vi "HexCenterFinder6Points.vi"() -> ()   [LabVIEW 2019]
uses:
  <vilib>/userDefined/High Color/IMAQdx.ctl
  <vilib>/vision/NI_Vision_Development_Module.lvlib
panel:
  in  "VisibleCorners":bool
  in  "AdjustCamera":T1={"+Y"=FALSE, "-Z"=FALSE, "Done"=FALSE, "+Z"=FALSE, "-Y"=FALSE, "-X"=FALSE, "+X"=FALSE, "MoveXYBy(mm)"=0.25, "MoveZBy(mm)"=0.1} {"MoveZBy(mm)" format="%#_13g"}
  out "CameraGcode":string
  out "Gcode":string
  out "Image":T2(plugin-control)
  in  "SiPatternLocations":path=path "C:/Users/TTUHEP/Documents/LabVIEW/Data/AssemblyIO_logs/Si2Fiducials.txt"
  out "Dev":dbl
  in  "YoffsetPCB":dbl format="%#_13g"
  in  "XoffsetPCB":dbl format="%#_13g"
  in  "Position1?":bool=TRUE
  in  "Yoffset":dbl format="%#_13g"
  in  "Xoffset":dbl=165.962 format="%#_13g"
  out "Output XYZU":string
  in  "PCBEdges":path=path "C:/Users/TTUHEP/Documents/LabVIEW/Data/AssemblyIO_logs/PCB1_4Points.txt"
  in  "SiNoPatternCorners":path=path "C:/Users/TTUHEP/Documents/LabVIEW/Data/AssemblyIO_logs/Si2Corners.txt"
  in  "Component":T3(ring)
  in  "BasePlateEdges":path=path "C:/Users/TTUHEP/Documents/LabVIEW/Data/AssemblyIO_logs/Baseplate1CuPoints.txt"
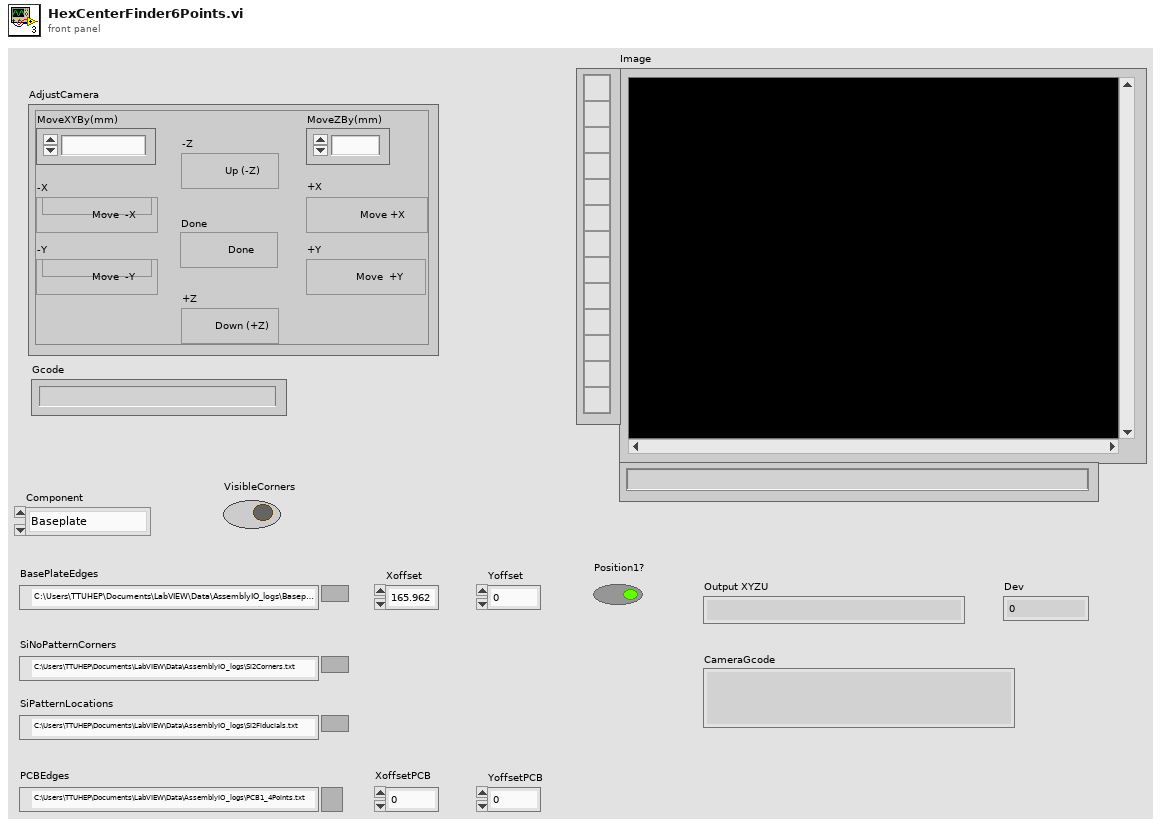
[diagram p1: front panel]
types:
  T1 = cluster{"+Y":bool, "-Z":bool, "Done":bool, "+Z":bool, "-Y":bool, "-X":bool, "+X":bool, "MoveXYBy(mm)":dbl, "MoveZBy(mm)":dbl}
  T2 = typedef "IMAQ Image.ctl" = refnum<image>
  T3 = enum16{"Baseplate", "SiNoPattern", "SiPattern", "PCB"}
  T4 = typedef "IMAQdx.ctl" = refnum<k21>
  T5 = typedef "IMAQ Point" = cluster{"X":sgl, "Y":sgl}
  T6 = enum16{"Left Button", "Center Button", "Right Button", "Window Close"}
  T7 = enum16{"open", "replace", "create", "open or create", "replace or create", "replace or create with confirmation"}
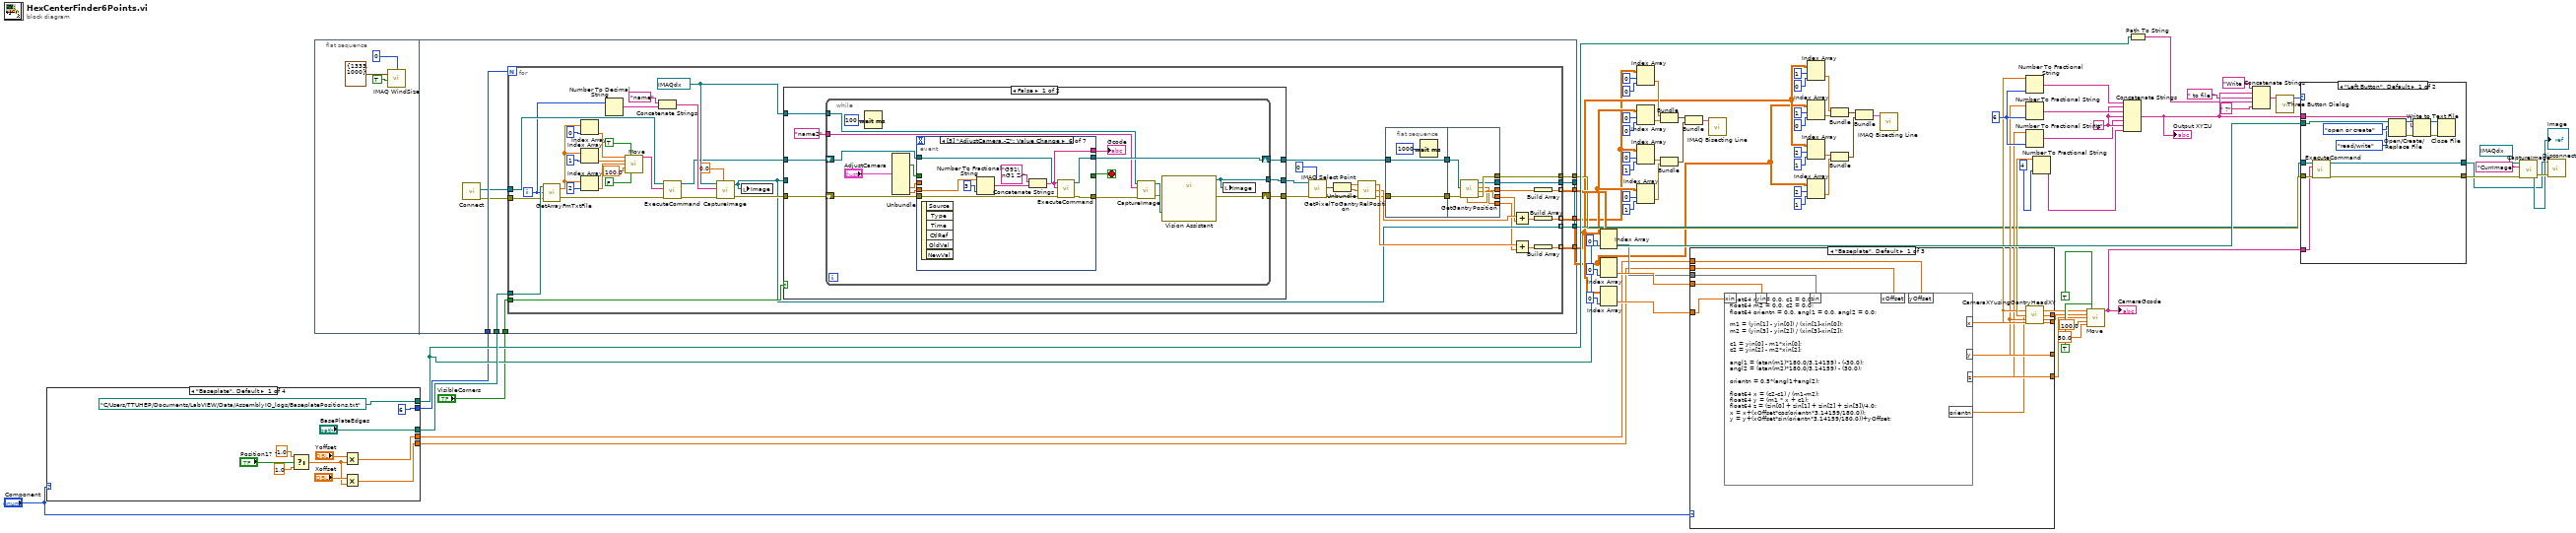
[diagram p0: block diagram]
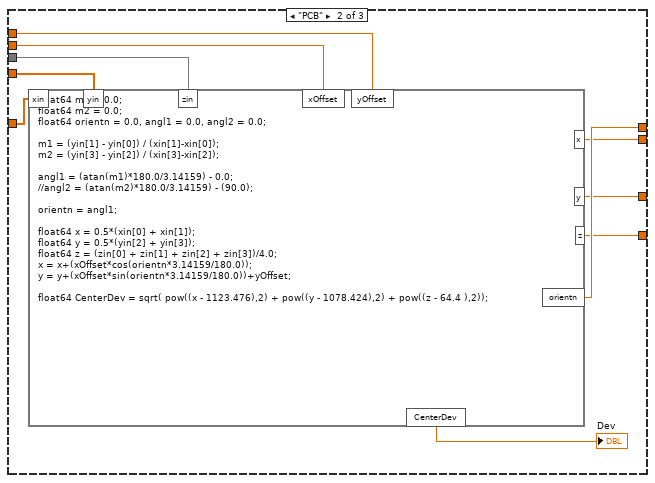
[diagram p2: hidden frame]
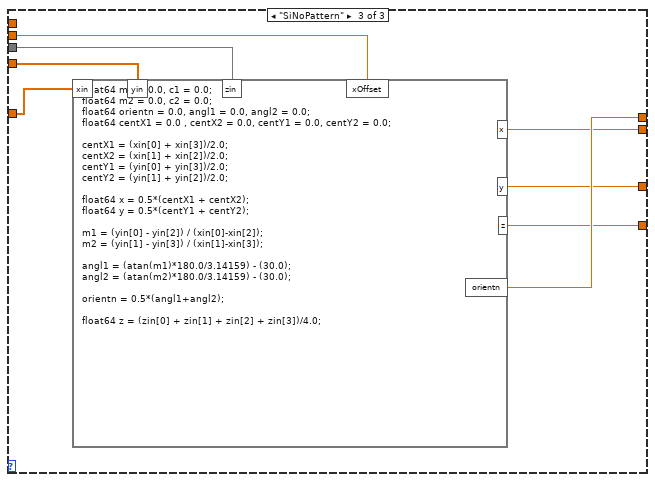
[diagram p3: hidden frame]
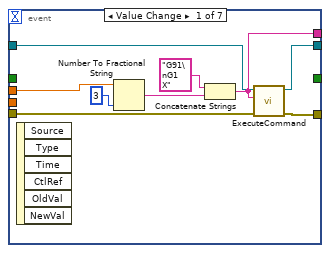
[diagram p5: hidden frame]
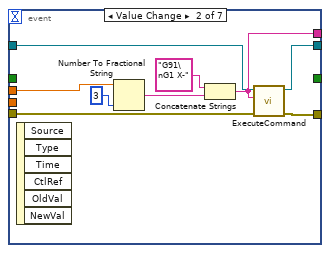
[diagram p6: hidden frame]
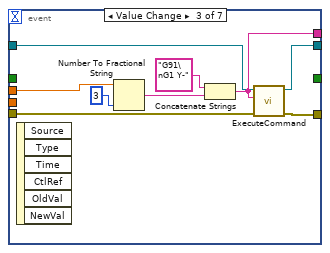
[diagram p7: hidden frame]
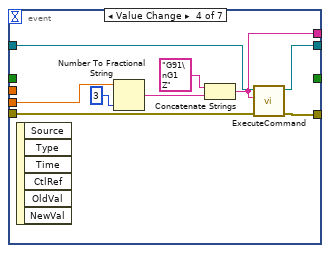
[diagram p8: hidden frame]
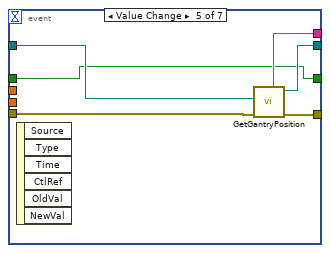
[diagram p9: hidden frame]
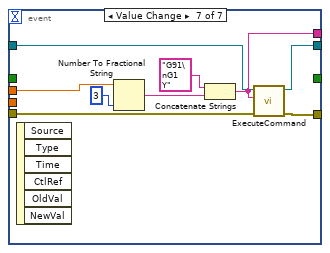
[diagram p10: hidden frame]
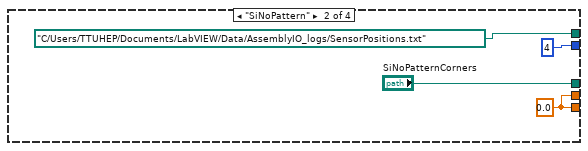
[diagram p12: hidden frame]
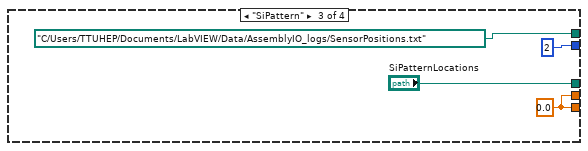
[diagram p13: hidden frame]
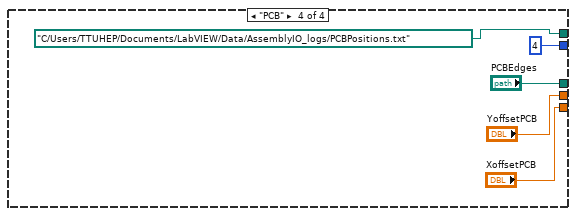
[diagram p14: hidden frame]
diagram:
  w76 = "\t"
  w73 = i16 6 ("width (-)")
  n1 = case shown="\"Baseplate\", Default" "Component" {
    tunnel: ["BasePlateEdges" "SiNoPatternCorners" "SiPatternLocations" "PCBEdges"] -> w79
    tunnel: [path "C:/Users/TTUHEP/Documents/LabVIEW/Data/AssemblyIO_logs/BaseplatePositions.txt" ("OutFile") path "C:/Users/TTUHEP/Documents/LabVIEW/Data/AssemblyIO_logs/SensorPositions.txt" ("OutFile") path "C:/Users/TTUHEP/Documents/LabVIEW/Data/AssemblyIO_logs/SensorPositions.txt" ("OutFile") path "C:/Users/TTUHEP/Documents/LabVIEW/Data/AssemblyIO_logs/PCBPositions.txt" ("OutFile")] -> w64
    tunnel: [w82 w92 w96 "YoffsetPCB"] -> w54
    tunnel: [w81 w92 w96 "XoffsetPCB"] -> w53
    tunnel: [6 4 2 4] -> w40
    frame "Baseplate", Default {
      n2 = Select(t=-1.0, s="Position1?", f=1.0 ("t")) -> (s? t:f=w83:dbl)
      n3 = Multiply(x="Yoffset", y=w83) -> (x*y=w82:dbl)
      n4 = Multiply(x="Xoffset", y=w83) -> (x*y=w81:dbl)
    }
    frame "SiNoPattern" {
      w92 = 0.0 ("YoffsetPCB")
    }
    frame "SiPattern" {
      w96 = 0.0 ("XoffsetPCB")
    }
    frame "PCB" {
    }
  }
  n5 = flat-sequence {
    tunnel: w40 -> [w117]
    tunnel: w79 -> [w116]
    tunnel: [w115] -> w38
    tunnel: [w114] -> w36
    tunnel: [w111] -> _
    tunnel: [w110] -> w62
    tunnel: [w109] -> w1
    tunnel: [w108] -> w2
    tunnel: "VisibleCorners" -> [w107]
    frame #0 {
      n6 = call "IMAQ WindSize"("Scrollbars? (N)"=TRUE, "Width & Height"=cluster{"Width":i32, "Height":i32} {"Width"=1333, "Height"=1000}, "Window Number"=0) -> ()  [unwired: 3 in, 3 out]
    }
    frame #1 {
      n7 = call "Connect.vi"() -> ("error out"=w113:errorcluster, "controller"=w112:refnum<k24>)  [unwired: 10 in]
      n8 = for {
        N: w117 -> [_]
        tunnel: w116 -> [w162]
        tunnel: w112 -> [w155]
        tunnel: w113 -> [w154]
        tunnel: [w126] -> w115
        tunnel: [w123] -> w114
        tunnel: [w127] -> w111 mode=indexing
        tunnel: [w148] -> w110 mode=indexing
        tunnel: [w142] -> w109 mode=indexing
        tunnel: [w141] -> w108 mode=indexing
        tunnel: w107 -> [w128]
        i -> [w152]
        w133 = T4 "cam0" ("Camera")
        n9 = call "GetArrayFmTxtFile.vi"("error in"=w154, "LineNo."=w152, "TextFile"=w162) -> ("error out"=w153:errorcluster, "Array"=w163:dbl[])
        n10 = Index Array(array=w163, index=0) -> (element=w139:dbl)
        n11 = Index Array(array=w163, index=1) -> (element=w137:dbl)
        n12 = Index Array(array=w163, index=2) -> (element=w147:dbl)
        n13 = Number To Decimal String(number=w152) -> (decimal integer string=w151:string)  [unwired: 1 in]
        n14 = call "Move.vi"("X"=w139, "Absolute"=TRUE, "Y"=w137, "Z"=w147, "SpeedXY (mm/s)"=100.0, "Move Z first"=FALSE) -> ("Position Gcode"=w156:string)  [unwired: 9 in]
        n15 = Concatenate Strings("name" ("string"), w151) -> (w149:string)
        n16 = call "ExecuteCommand.vi"("error in (no error)"=w153, "Command Code"=w156, "controller in"=w155) -> ("error out"=w158:errorcluster, "controller out"=w132:refnum<k24>)  [unwired: 6 in, 1 out]
        n17 = call "CaptureImage.vi"("Camera"=w133, "Rotate (degrees)"=sgl 0.0, "ImageName"=w149, "error in (no error)"=w158) -> ("Image"=w127:T2, "error out"=w131:errorcluster)  [unwired: 3 in]
        n18 = local write "Image"(w127) -> ()
        n19 = case shown="False" w128 {
          tunnel: w133 -> [w182 _]
          tunnel: w132 -> [w181 w262]
          tunnel: w131 -> [w180 w263]
          tunnel: [w179 w261] -> w130
          tunnel: [w178 w262] -> w119
          tunnel: [w177 w263] -> w129
          tunnel: w127 -> [_ w261]
          frame False {
            n20 = while {
              shift-right: [w191] -> w177
              shift-left: w180 -> [w200]
              shift-right: [w198] -> w178
              shift-left: w181 -> [w199]
              tunnel: "name2" ("ImageName") -> [w193]
              tunnel: w182 -> [w194]
              tunnel: [w190] -> w179
              stop <- w196 stop-if-true
              n21 = Wait (ms)(milliseconds to wait=u32 100) -> ()  [unwired: 1 out]
              n22 = Unbundle("AdjustCamera") -> ("Done"=w186:bool, "MoveXYBy(mm)"=w184:dbl, "MoveZBy(mm)"=w185:dbl)  [unwired: 6 out]
              n23 = event shown="[5] \"AdjustCamera.-Z\": Value Change" {
                selector: _ -> [_ _ _ _ _ _ _]
                dyn-events: _ -> [_ _ _ _ _ _ _]
                timeout: _ -> [_ _ _ _ _ _ _]
                tunnel: w184 -> [w206 w210 w219 _ _ _ w252]
                tunnel: w200 -> [w205 w214 w223 w232 w241 w247 w256]
                tunnel: [w204 w213 w222 w229 w238 w246 w255] -> w192
                tunnel: w199 -> [w203 w215 w224 w233 w242 w248 w257]
                tunnel: [w202 w212 w221 w230 w240 w245 w254] -> w198
                tunnel: [w201 w211 w220 w231 w239 w244 w253] -> w197
                tunnel: [_ _ _ _ w237 _ _] -> w196
                tunnel: w185 -> [_ _ _ w228 _ w243 _]
                tunnel: w186 -> [_ _ _ _ w237 _ _]
                event "AdjustCamera.+X": Value Change {
                  n24 = event-data() -> ()  [unwired: 1 in, 6 out]
                  n25 = Number To Fractional String(number=w206, precision (6)=3) -> (F-format string=w209:string)  [unwired: 2 in]
                  n26 = Concatenate Strings("G91\nG1 X", w209) -> (w201:string)
                  n27 = call "ExecuteCommand.vi"("error in (no error)"=w205, "Command Code"=w201, "controller in"=w203) -> ("error out"=w204:errorcluster, "controller out"=w202:refnum<k24>)  [unwired: 6 in, 1 out]
                }
                event "AdjustCamera.-X": Value Change {
                  n28 = event-data() -> ()  [unwired: 1 in, 6 out]
                  n29 = Number To Fractional String(number=w210, precision (6)=3) -> (F-format string=w218:string)  [unwired: 2 in]
                  n30 = Concatenate Strings("G91\nG1 X-", w218) -> (w211:string)
                  n31 = call "ExecuteCommand.vi"("error in (no error)"=w214, "Command Code"=w211, "controller in"=w215) -> ("error out"=w213:errorcluster, "controller out"=w212:refnum<k24>)  [unwired: 6 in, 1 out]
                }
                event "AdjustCamera.-Y": Value Change {
                  n32 = event-data() -> ()  [unwired: 1 in, 6 out]
                  n33 = Number To Fractional String(number=w219, precision (6)=3) -> (F-format string=w227:string)  [unwired: 2 in]
                  n34 = Concatenate Strings("G91\nG1 Y-", w227) -> (w220:string)
                  n35 = call "ExecuteCommand.vi"("error in (no error)"=w223, "Command Code"=w220, "controller in"=w224) -> ("error out"=w222:errorcluster, "controller out"=w221:refnum<k24>)  [unwired: 6 in, 1 out]
                }
                event "AdjustCamera.+Z": Value Change {
                  n36 = event-data() -> ()  [unwired: 1 in, 6 out]
                  n37 = Number To Fractional String(number=w228, precision (6)=3) -> (F-format string=w236:string)  [unwired: 2 in]
                  n38 = Concatenate Strings("G91\nG1 Z", w236) -> (w231:string)
                  n39 = call "ExecuteCommand.vi"("error in (no error)"=w232, "Command Code"=w231, "controller in"=w233) -> ("error out"=w229:errorcluster, "controller out"=w230:refnum<k24>)  [unwired: 6 in, 1 out]
                }
                event "AdjustCamera.Done": Value Change {
                  n40 = event-data() -> ()  [unwired: 1 in, 6 out]
                  n41 = call "GetGantryPosition.vi"("error in (no error)"=w241, "Controller In"=w242) -> ("error out"=w238:errorcluster, "controller out"=w240:refnum<k24>, "Position_XYZ"=w239:string)  [unwired: 3 in, 4 out]
                }
                event "AdjustCamera.-Z": Value Change {
                  n42 = event-data() -> ()  [unwired: 1 in, 6 out]
                  n43 = Number To Fractional String(number=w243, precision (6)=3) -> (F-format string=w251:string)  [unwired: 2 in]
                  n44 = Concatenate Strings("G91\nG1 Z-", w251) -> (w244:string)
                  n45 = call "ExecuteCommand.vi"("error in (no error)"=w247, "Command Code"=w244, "controller in"=w248) -> ("error out"=w246:errorcluster, "controller out"=w245:refnum<k24>)  [unwired: 6 in, 1 out]
                }
                event "AdjustCamera.+Y": Value Change {
                  n46 = event-data() -> ()  [unwired: 1 in, 6 out]
                  n47 = Number To Fractional String(number=w252, precision (6)=3) -> (F-format string=w260:string)  [unwired: 2 in]
                  n48 = Concatenate Strings("G91\nG1 Y", w260) -> (w253:string)
                  n49 = call "ExecuteCommand.vi"("error in (no error)"=w256, "Command Code"=w253, "controller in"=w257) -> ("error out"=w255:errorcluster, "controller out"=w254:refnum<k24>)  [unwired: 6 in, 1 out]
                }
              }
              "Gcode" <- w197
              n50 = call "CaptureImage.vi"("Camera"=w194, "ImageName"=w193, "error in (no error)"=w192) -> ("Image"=w189:T2, "error out"=w188:errorcluster)  [unwired: 4 in]
              n51 = call "Vision Assistant"("Image In"=w189, "error in"=w188) -> ("Image Out"=w190:T2, "error out"=w191:errorcluster)  [unwired: 24 in]
              n52 = local write "Image"(w190) -> ()
            }
          }
          frame True {
          }
        }
        n53 = call "IMAQ Select Point"("Window Number (0...15)"=0, "error in (no error)"=w129, "Image In"=w130) -> ("error out"=w143:errorcluster, "Point"=w146:T5)  [unwired: 5 in, 2 out]
        n54 = Unbundle(w146) -> ("X"=w145:sgl, "Y"=w144:sgl)
        n55 = call "GetPixelToGantryRelPosition.vi"("error in (no error)"=w143, "PixelY"=w144, "PixelX"=w145) -> ("error out"=w121:errorcluster, "YmmRelGH"=w136:dbl, "XmmRelGH"=w140:dbl)
        n56 = flat-sequence {
          tunnel: w121 -> [w168]
          tunnel: [w168] -> w120
          tunnel: w119 -> [w167]
          tunnel: [w167] -> w118
          tunnel: [w176] -> w126
          tunnel: [w175] -> w125
          tunnel: [w174] -> w124
          tunnel: [w173] -> w123
          tunnel: [w172] -> w122
          tunnel: w120 -> [w171]
          tunnel: w118 -> [w170]
          frame #0 {
            n57 = Wait (ms)(milliseconds to wait=u32 1000) -> ()  [unwired: 1 out]
          }
          frame #1 {
            n58 = call "GetGantryPosition.vi"("error in (no error)"=w171, "Controller In"=w170) -> ("error out"=w176:errorcluster, "Position Y"=w175:dbl, "Position X"=w174:dbl, "controller out"=w173:refnum<k24>, "Position Z"=w172:dbl)  [unwired: 3 in, 2 out]
          }
        }
        n59 = Add(x=w136, y=w125) -> (x+y=w135:dbl)
        n60 = Add(x=w140, y=w124) -> (x+y=w138:dbl)
        n61 = Build Array(w122) -> (w148:dbl[])
        n62 = Build Array(w135) -> (w142:dbl[])
        n63 = Build Array(w138) -> (w141:dbl[])
      }
    }
  }
  n64 = Index Array(array=w62, index (col)=0 ("disabled index (col)")) -> (element=w57:dbl[])  [unwired: 1 in]
  n65 = Index Array(array=w1, index (col)=0 ("disabled index (col)")) -> (element=w58:dbl[])  [unwired: 1 in]
  n66 = Index Array(array=w2, index (col)=0 ("disabled index (col)")) -> (element=w59:dbl[])  [unwired: 1 in]
  n67 = Index Array(array=w1, index (row)=0 ("disabled index (row)"), index (col)=0 ("disabled index (col)")) -> (element=w24:dbl)
  n68 = Index Array(array=w2, index (row)=0 ("disabled index (row)"), index (col)=0 ("disabled index (col)")) -> (element=w23:dbl)
  n69 = Index Array(array=w1, index (row)=0 ("disabled index (row)"), index (col)=1 ("disabled index (col)")) -> (element=w22:dbl)
  n70 = Index Array(array=w2, index (row)=0 ("disabled index (row)"), index (col)=1 ("disabled index (col)")) -> (element=w21:dbl)
  n71 = Bundle(w24, w23) -> (w20:cluster{dbl, dbl})  [unwired: 1 in]
  n72 = Bundle(w22, w21) -> (w19:cluster{dbl, dbl})  [unwired: 1 in]
  n73 = Bundle(w20, w19) -> (w18:cluster{cluster{dbl, dbl}, cluster{dbl, dbl}})  [unwired: 1 in]
  n74 = case shown="\"Baseplate\", Default" "Component" {
    tunnel: w59 -> [w272 w282 w290]
    tunnel: w58 -> [w271 w281 w289]
    tunnel: w57 -> [w270 w280 w288]
    tunnel: w53 -> [w269 w279 w287]
    tunnel: [w268 w278 w286] -> w56
    tunnel: [w267 w277 w285] -> w45
    tunnel: [w266 w276 w284] -> w44
    tunnel: [w265 w275 w283] -> w41
    tunnel: w54 -> [w264 w274 _]
    frame "Baseplate", Default {
      n75 = formula code="float64 m1 = 0.0, c1 = 0.0;\nfloat64 m2 = 0.0, c2 = 0.0;\nfloat64 orientn = 0.0, angl1 = 0.0, angl2 = 0.0;\n\nm1 = (yin[1] - yin[0]) / (xin[1]-xin[0]);\nm2 = (yin[3] - yin[2]) / (xin[3]-xin[2]);\n\nc1 = yin[0] - m1*xin[0];\nc2 = yin[2] - m2*xin[2];\n\nangl1 = (atan(m1)*180.0/3.14159) - (-30.0);\nangl2 = (atan(m2)*180.0/3.14159) - (30.0);\n\norientn = 0.5*(angl1+angl2);\n\nfloat64 x = (c2-c1) / (m1-m2);\nfloat64 y = (m1 * x + c1);\nfloat64 z = (zin[0] + zin[1] + zin[2] + zin[3])/4.0;\nx = x+(xOffset*cos(orientn*3.14159/180.0));\ny = y+(xOffset*sin(orientn*3.14159/180.0))+yOffset;"("xin"=w272, "yin"=w271, "zin"=w270, "xOffset"=w269, "yOffset"=w264) -> ("orientn"=w268:dbl, "x"=w267:dbl, "y"=w266:dbl, "z"=w265:dbl)
    }
    frame "PCB" {
      n76 = formula code="float64 m1 = 0.0;\nfloat64 m2 = 0.0;\nfloat64 orientn = 0.0, angl1 = 0.0, angl2 = 0.0;\n\nm1 = (yin[1] - yin[0]) / (xin[1]-xin[0]);\nm2 = (yin[3] - yin[2]) / (xin[3]-xin[2]);\n\nangl1 = (atan(m1)*180.0/3.14159) - 0.0;\n//angl2 = (atan(m2)*180.0/3.14159) - (90.0);\n\norientn = angl1;\n\nfloat64 x = 0.5*(xin[0] + xin[1]);\nfloat64 y = 0.5*(yin[2] + yin[3]);\nfloat64 z = (zin[0] + zin[1] + zin[2] + zin[3])/4.0;\nx = x+(xOffset*cos(orientn*3.14159/180.0));\ny = y+(xOffset*sin(orientn*3.14159/180.0))+yOffset;\n\nfloat64 CenterDev = sqrt( pow((x - 1123.476),2) + pow((y - 1078.424),2) + pow((z - 64.4 ),2));"("xin"=w282, "yin"=w281, "zin"=w280, "xOffset"=w279, "yOffset"=w274) -> ("orientn"=w278:dbl, "x"=w277:dbl, "y"=w276:dbl, "z"=w275:dbl, "CenterDev"=→"Dev":dbl)
    }
    frame "SiNoPattern" {
      n77 = formula code="float64 m1 = 0.0, c1 = 0.0;\nfloat64 m2 = 0.0, c2 = 0.0;\nfloat64 orientn = 0.0, angl1 = 0.0, angl2 = 0.0;\nfloat64 centX1 = 0.0 , centX2 = 0.0, centY1 = 0.0, centY2 = 0.0;\n\ncentX1 = (xin[0] + xin[3])/2.0;\ncentX2 = (xin[1] + xin[2])/2.0;\ncentY1 = (yin[0] + yin[3])/2.0;\ncentY2 = (yin[1] + yin[2])/2.0;\n\nfloat64 x = 0.5*(centX1 + centX2); \nfloat64 y = 0.5*(centY1 + centY2);\n\nm1 = (yin[0] - yin[2]) / (xin[0]-xin[2]);\nm2 = (yin[1] - yin[3]) / (xin[1]-xin[3]);\n\nangl1 = (atan(m1)*180.0/3.14159) - (30.0);\nangl2 = (atan(m2)*180.0/3.14159) - (30.0);\n\norientn = 0.5*(angl1+angl2);\n\nfloat64 z = (zin[0] + zin[1] + zin[2] + zin[3])/4.0;"("xin"=w290, "yin"=w289, "zin"=w288, "xOffset"=w287) -> ("orientn"=w286:dbl, "x"=w285:dbl, "y"=w284:dbl, "z"=w283:dbl)
    }
  }
  n78 = call "IMAQ Bisecting Line"("Line 1"=w18) -> ()  [unwired: 9 in, 2 out]
  n79 = Index Array(array=w2, index (row)=1 ("disabled index (row)"), index (col)=0 ("disabled index (col)")) -> (element=w9:dbl)
  n80 = Index Array(array=w1, index (row)=1 ("disabled index (row)"), index (col)=0 ("disabled index (col)")) -> (element=w8:dbl)
  n81 = Index Array(array=w2, index (row)=2 ("disabled index (row)"), index (col)=1 ("disabled index (col)")) -> (element=w7:dbl)
  n82 = Index Array(array=w1, index (row)=2 ("disabled index (row)"), index (col)=1 ("disabled index (col)")) -> (element=w6:dbl)
  n83 = Bundle(w9, w8) -> (w5:cluster{dbl, dbl})  [unwired: 1 in]
  n84 = Bundle(w7, w6) -> (w4:cluster{dbl, dbl})  [unwired: 1 in]
  n85 = Bundle(w5, w4) -> (w3:cluster{cluster{dbl, dbl}, cluster{dbl, dbl}})  [unwired: 1 in]
  n86 = call "IMAQ Bisecting Line"("Line 1"=w3) -> ()  [unwired: 9 in, 2 out]
  n87 = Number To Fractional String(number=w45, precision (6)=w73) -> (F-format string=w78:string)  [unwired: 2 in]
  n88 = Number To Fractional String(number=w44, precision (6)=w73) -> (F-format string=w77:string)  [unwired: 2 in]
  n89 = Number To Fractional String(number=w41, precision (6)=w73) -> (F-format string=w72:string)  [unwired: 2 in]
  n90 = call "CameraXYusingGantryHeadXY.vi"("GantryY"=w44, "GantryX"=w45) -> ("CamY"=w42:dbl, "CamX"=w43:dbl)
  n91 = Number To Fractional String(number=w56, precision (6)=i16 4 ("width (-)")) -> (F-format string=w74:string)  [unwired: 2 in]
  n92 = call "Move.vi"("X"=w43, "Absolute"=TRUE, "Y"=w42, "Z"=w41, "SpeedXY (mm/s)"=100.0, "SpeedZ (mm/s)"=50.0, "Move Z first"=TRUE) -> ("Position Gcode"=w37:string)  [unwired: 8 in]
  "CameraGcode" <- w37
  n93 = Concatenate Strings(w78, w76, w77, w76, w72, w76, w74) -> (w70:string)
  "Output XYZU" <- w70
  n94 = Path To String(path=w64) -> (string=w68:string)
  n95 = Concatenate Strings("Write ", w70, " to file ", w68, " ?" ("string")) -> (w66:string)
  n96 = call <vilib>:"Three Button Dialog.vi"("message"=w66) -> ("Which Button?"=w65:T6)  [unwired: 10 in]
  n97 = case shown="\"Left Button\", Default" w65 {
    tunnel: w70 -> [w297 _]
    tunnel: w64 -> [w296 _]
    tunnel: w38 -> [w295 w305]
    tunnel: w37 -> [w294 _]
    tunnel: w36 -> [w293 w304]
    tunnel: [w292 w305] -> w35
    tunnel: [w291 w304] -> w34
    frame "Left Button", Default {
      n98 = call "ExecuteCommand.vi"("error in (no error)"=w295, "Command Code"=w294, "controller in"=w293) -> ("error out"=w292:errorcluster, "controller out"=w291:refnum<k24>)  [unwired: 6 in, 1 out]
      n99 = Open/Create/Replace File(file path (use dialog)=w296, operation (0:open)=T7."open or create", access (0:read/write)=enum16{"read/write", "read-only", "write-only"}."read/write") -> (refnum out=w303:refnum<file>, error out=w300:errorcluster)  [unwired: 3 in, 1 out]
      n100 = Write to Text File(file (use dialog)=w303, text=w297, error in=w300) -> (refnum out=w298:refnum<file>, error out=w299:errorcluster)  [unwired: 1 in, 1 out]
      n101 = Close File(refnum=w298, error in=w299) -> ()  [unwired: 2 out]
    }
    frame "Center Button" {
    }
  }
  n102 = call "CaptureImage.vi"("Camera"=T4 "cam0", "ImageName"="CurrImage", "error in (no error)"=w35) -> ("Image"=→"Image":T2, "error out"=w48:errorcluster)  [unwired: 4 in]
  n103 = call "Disconnect.vi"("error in (no error)"=w48, "controller"=w34) -> ()  [unwired: 9 in, 1 out]
